vi "Copy Package.vi"(8 "error in (no error)":errorcluster, 11 "PostBuildSupport in":refnum<class "PostBuildSupport (2013).lvclass">) -> (0 "error out":errorcluster, 3 "PostBuildSupport out":refnum<class "PostBuildSupport (2013).lvclass">)   [LabVIEW 2016, in "PostBuildSupport (2013).lvclass"]
uses:
  PostBuildSupport (2013).lvclass
  PostBuildSupport (2013).lvclass/PostBuildSupport (2013).ctl
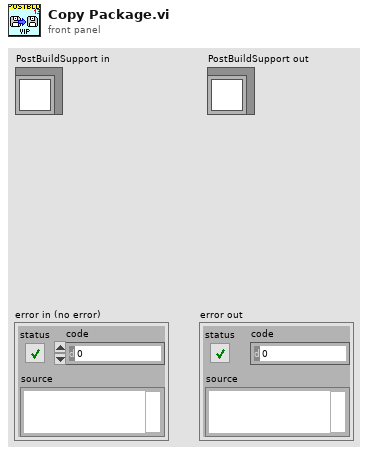
[diagram p1: front panel]
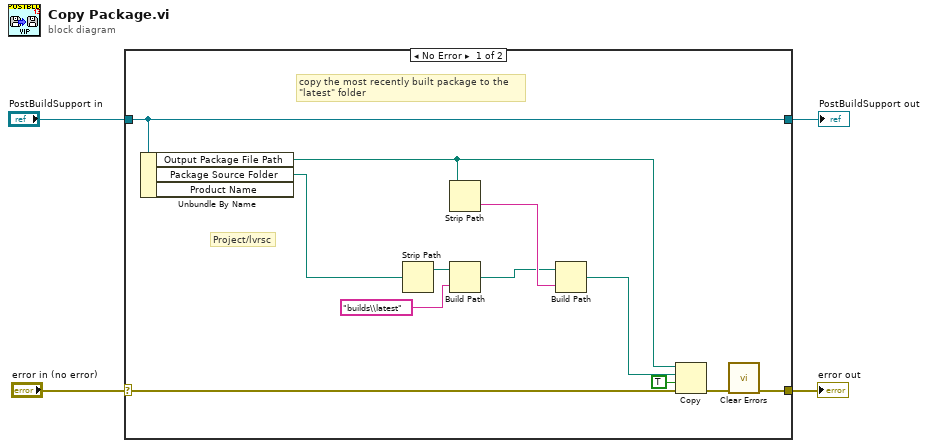
[diagram p0: block diagram]
diagram:
  n1 = case shown="No Error" "error in (no error)" {
    selector: "error in (no error)" -> [w10 w18]
    tunnel: [w7 w18] -> w4
    tunnel: "PostBuildSupport in" -> [w9 w17]
    tunnel: [w9 w17] -> w1
    frame No Error {
      # "Project/lvrsc"
      # "copy the most recently built package to the \n\"latest\" folder"
      n2 = Unbundle By Name(w9) -> ("Output Package File Path"=w11:path, "Package Source Folder"=w12:path)  [unwired: 1 out]
      n3 = Strip Path(path=w12) -> (stripped path=w16:path)  [unwired: 1 out]
      n4 = Strip Path(path=w11) -> (name=w15:string)  [unwired: 1 out]
      n5 = Build Path(base path=w16, name or relative path="builds\\latest") -> (appended path=w6:path)
      n6 = Build Path(base path=w6, name or relative path=w15) -> (appended path=w14:path)
      n7 = Copy(8:w10, 9:TRUE ("overwrite (F)"), 10:w14, 11:w11) -> (0:w8:errorcluster)  [unwired: 1 in, 2 out]
      n8 = call <vilib>:"Clear Errors.vi"("error in (no error)"=w8) -> ("error out"=w7:errorcluster)  [unwired: 5 in, 1 out]
    }
    frame Error {
    }
  }
  "error out" <- w4
  "PostBuildSupport out" <- w1
